vi "Exemple_Preprocessing_normalize.vi"() -> ()   [LabVIEW 2020]
panel:
  out "Data":T1
  out "error out":errorcluster
  in  "X":string[][](array[string])=[["4", "1", "2", "2"], ["1", "3", "9", "3"], ["5", "7", "5", "1"]]
  in  "error in":errorcluster caption="entrée d'erreur"
  in  "normalize":T2={"norm"="l2", "axis"=1, "copy"=TRUE, "Returns"="X"}
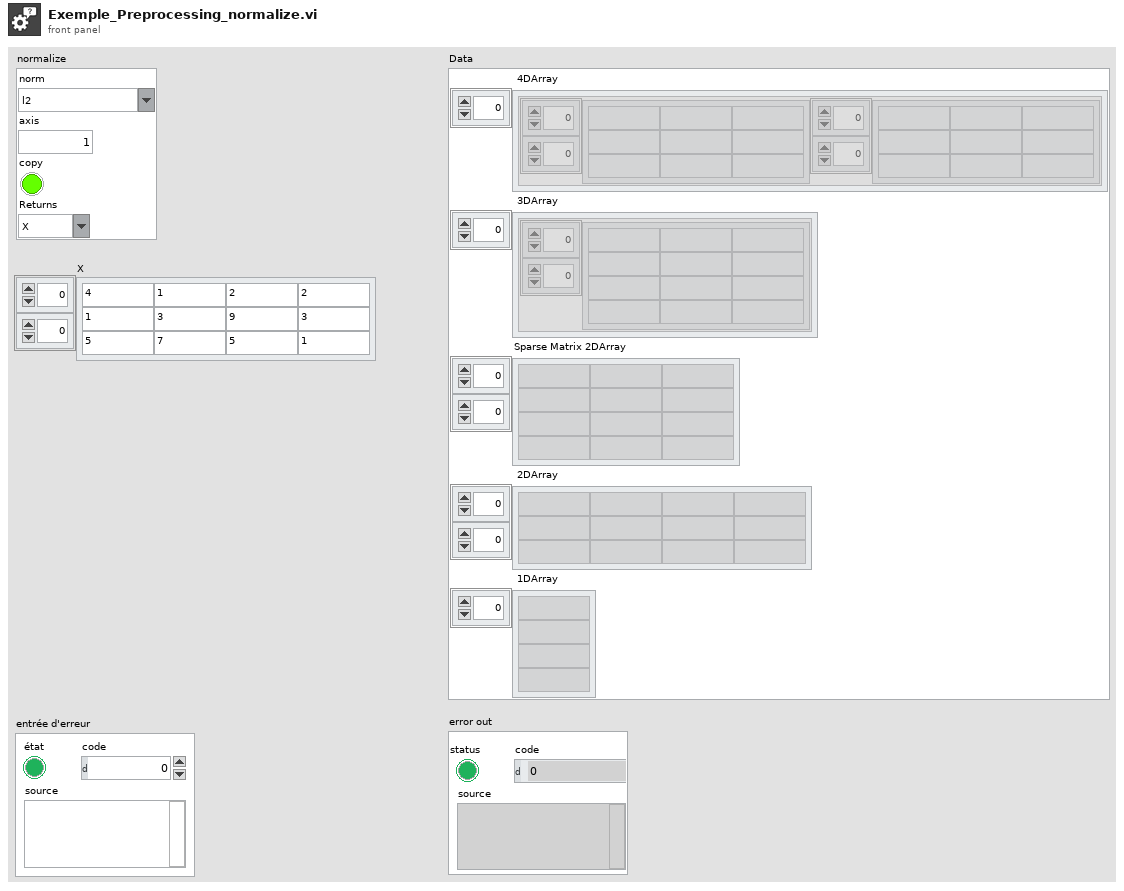
[diagram p1: front panel]
types:
  T1 = cluster{" 4DArray":cluster{"1":string[][], "2":string[][]}[], " 3DArray":cluster{"Tableau":string[][]}[], "Sparse Matrix 2DArray":string[][], " 2DArray":string[][], " 1DArray":string[]}
  T2 = cluster{"norm":string, "axis":i32, "copy":bool, "Returns":string}
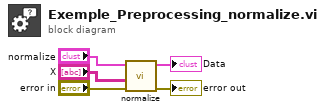
[diagram p0: block diagram]
diagram:
  n1 = call "normalize.vi"("error in"="error in", "X"="X", "normalize"="normalize") -> ("error out"=→"error out":errorcluster, "Data"=→"Data":T1)  [unwired: 7 in]
